vi "simulation.vi"(0 "Angle":dbl[](array[numeric]), 1 "dt":dbl=0.01, 2 "Map Data":T1, 5 "R dir":dbl(slide) scale=3.2..-3.2, 7 "Robot Radius":dbl=6.0, 9 "R pos":dbl[](array[numeric])=[0.0, 0.0], 11 "LRF range":dbl=40.0, 12 "w":dbl=2.0, 13 "LRF offset":dbl=5.0, 14 "v":dbl=2.0) -> (3 "Mapped Data Visual out":T2(graph), 4 "Robot pos new":dbl[](array[numeric]), 10 "Robot dir new":dbl(slide) scale=3.2..-3.2, 15 "LRF":dbl[](array[numeric]))   [LabVIEW 2009]
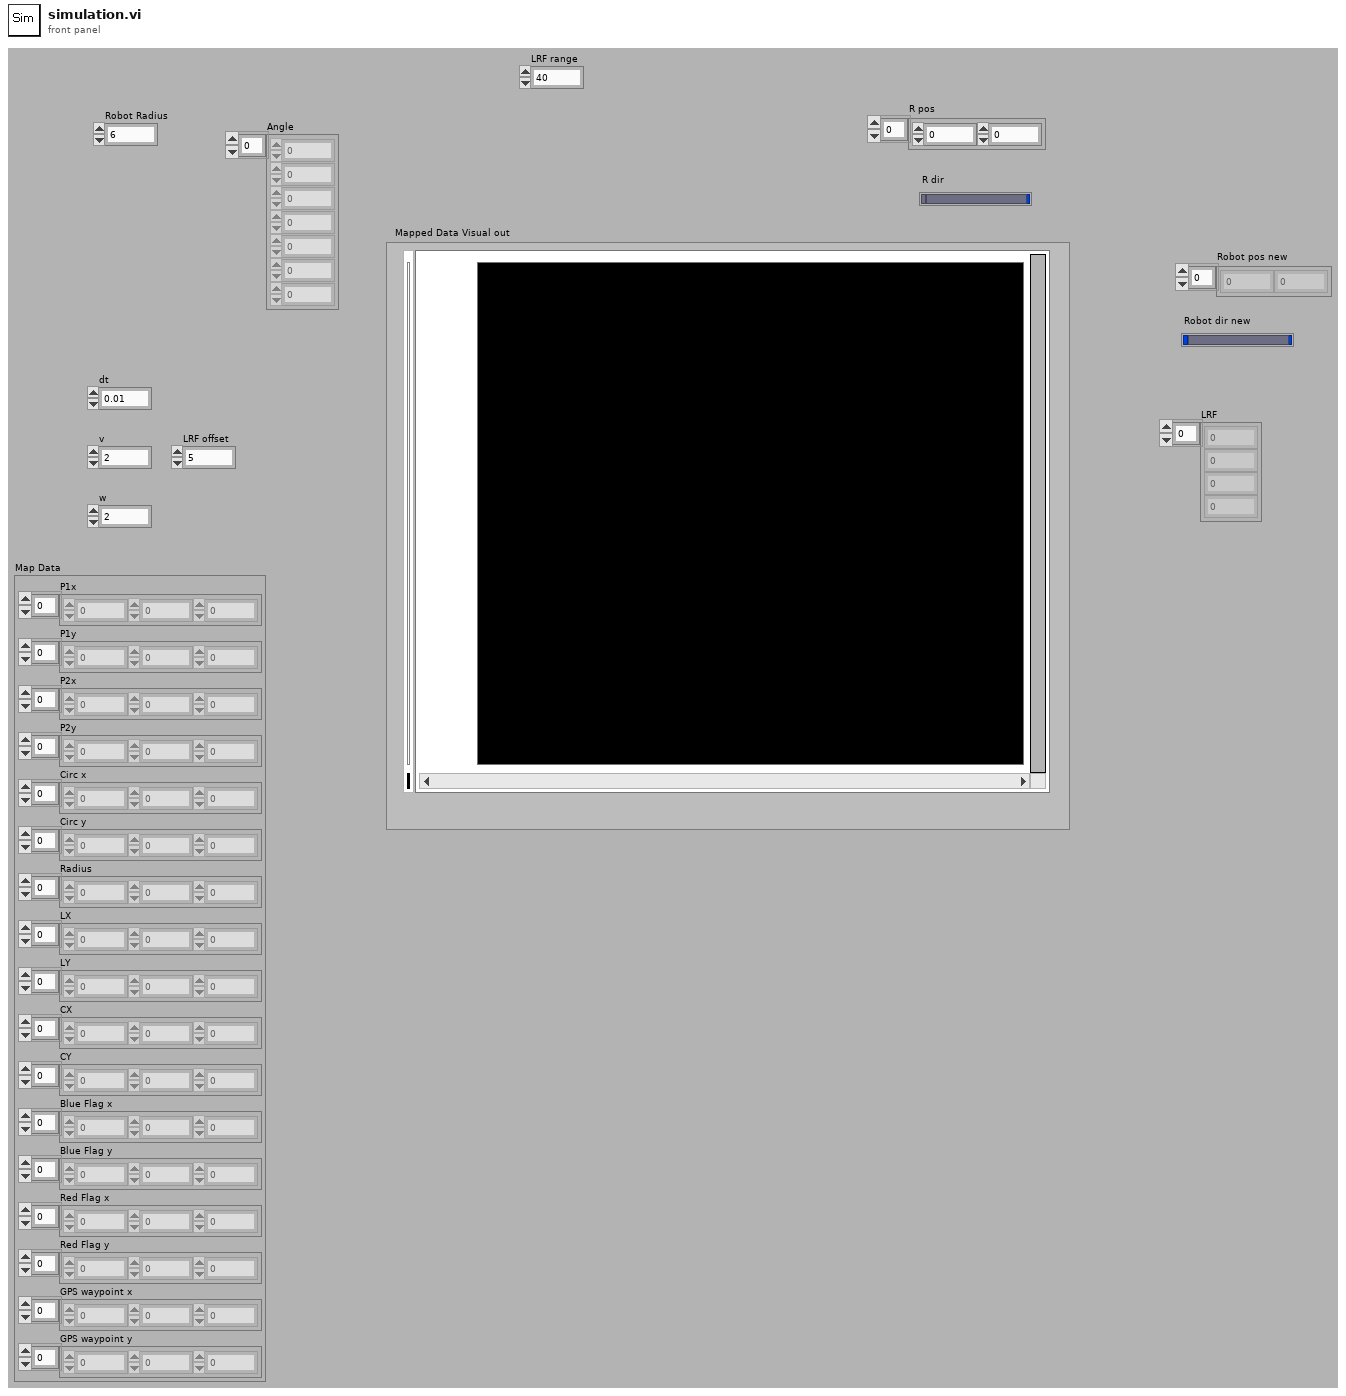
[diagram p1: front panel]
types:
  T1 = cluster{"P1x":dbl[], "P1y":dbl[], "P2x":dbl[], "P2y":dbl[], "Circ x":dbl[], "Circ y":dbl[], "Radius":dbl[], "LX":dbl[], "LY":dbl[], "CX":dbl[], "CY":dbl[], "Blue Flag x":dbl[], "Blue Flag y":dbl[], "Red Flag x":dbl[], "Red Flag y":dbl[], "GPS waypoint x":dbl[], "GPS waypoint y":dbl[]}
  T2 = cluster{cluster{dbl[], dbl[]}, "output cluster":cluster{dbl[], dbl[]}, cluster{dbl[], dbl[]}, cluster{dbl[], dbl[]}, cluster{dbl[], dbl[]}, cluster{dbl[], dbl[]}, cluster{dbl[], dbl[]}}
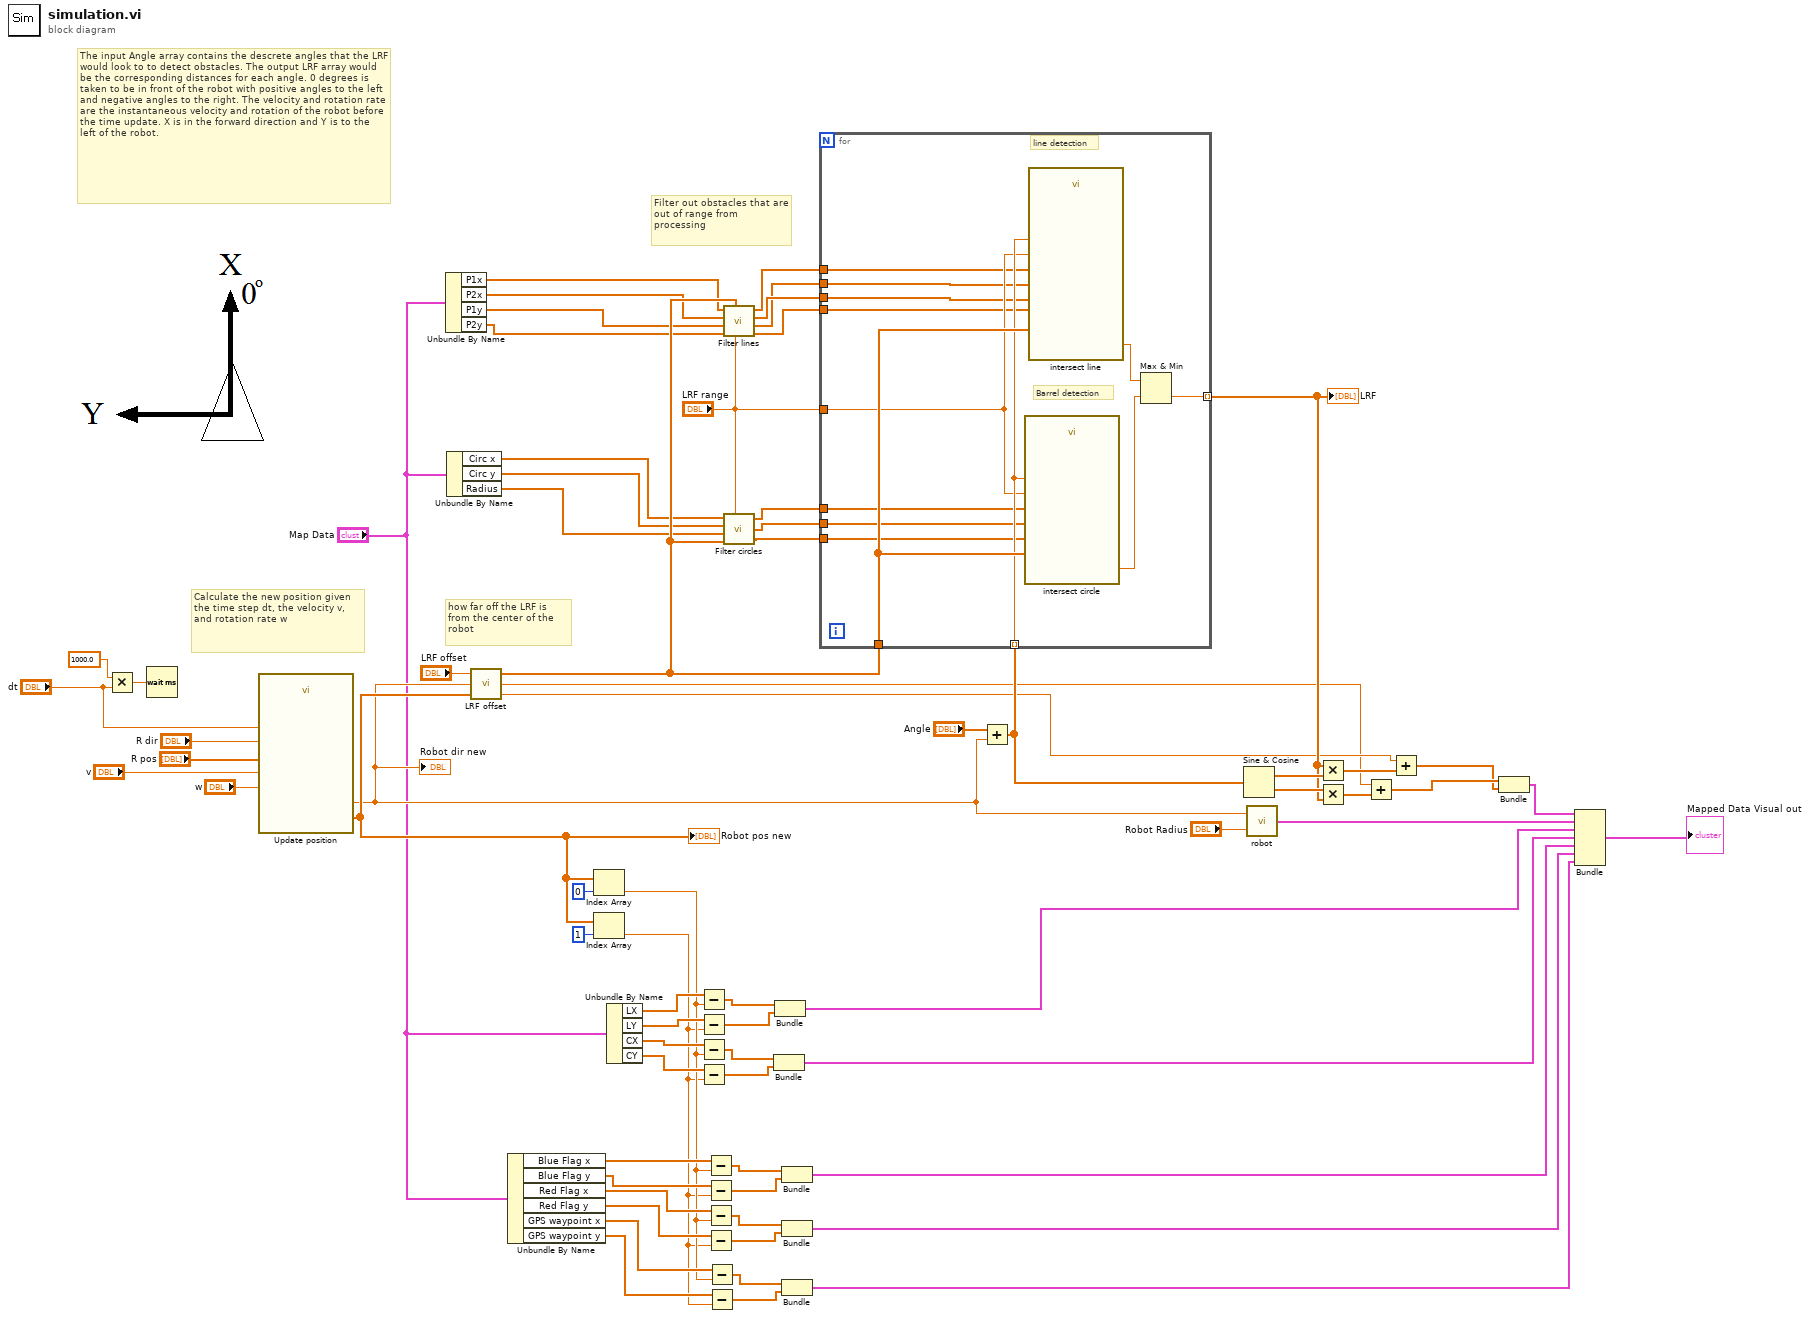
[diagram p0: block diagram]
diagram:
  # "how far off the LRF is from the center of the robot"
  # "The input Angle array contains the descrete angles that the LRF would look to to detect obstacles. The output LRF array would be the corresponding distances for each angle. 0 degrees is taken to be in front of the robot with positive angles to the left and negative angles to the right. The velocity and rotation rate are the instantaneous velocity and rotation of the robot before the time update. X is in the forward direction and Y is to the left of the robot."
  # "Filter out obstacles that are out of range from processing"
  # "Calculate the new position given the time step dt, the velocity v, and rotation rate w"
  n1 = Multiply(x=1000.0 ("y"), y="dt") -> (x*y=w66:dbl)
  n2 = Wait (ms)(milliseconds to wait=w66) -> ()  [unwired: 1 out]
  n3 = call "Update position.vi"("R pos"="R pos", "R dir"="R dir", "dt"="dt", "v"="v", "w"="w") -> ("R pos new"=w30:dbl[], "R dir new"=w20:dbl)
  "Robot pos new" <- w30
  "Robot dir new" <- w20
  n4 = Unbundle By Name("Map Data") -> ("P1x"=w37:dbl[], "P2x"=w36:dbl[], "P1y"=w35:dbl[], "P2y"=w34:dbl[])
  n5 = Unbundle By Name("Map Data") -> ("Circ x"=w40:dbl[], "Circ y"=w39:dbl[], "Radius"=w38:dbl[])
  n6 = call "LRF offset.vi"("Robot position"=w30, "Robot direction"=w20, "LRF offset"="LRF offset") -> ("Dy"=w43:dbl, "Dx"=w42:dbl, "LRF position"=w47:dbl[])
  n7 = Unbundle By Name("Map Data") -> ("Blue Flag x"=w15:dbl[], "Blue Flag y"=w14:dbl[], "Red Flag x"=w13:dbl[], "Red Flag y"=w12:dbl[], "GPS waypoint x"=w9:dbl[], "GPS waypoint y"=w8:dbl[])
  n8 = Index Array(array=w30, index=0) -> (element=w7:dbl)
  n9 = Index Array(array=w30, index=1) -> (element=w6:dbl)
  n10 = Unbundle By Name("Map Data") -> ("LX"=w33:dbl[], "LY"=w29:dbl[], "CX"=w28:dbl[], "CY"=w27:dbl[])
  n11 = Subtract(x=w33, y=w7) -> (x-y=w26:dbl[])
  n12 = Subtract(x=w29, y=w6) -> (x-y=w25:dbl[])
  n13 = Subtract(x=w28, y=w7) -> (x-y=w24:dbl[])
  n14 = Subtract(x=w27, y=w6) -> (x-y=w23:dbl[])
  n15 = Subtract(x=w15, y=w7) -> (x-y=w19:dbl[])
  n16 = Subtract(x=w14, y=w6) -> (x-y=w18:dbl[])
  n17 = Subtract(x=w13, y=w7) -> (x-y=w17:dbl[])
  n18 = Subtract(x=w12, y=w6) -> (x-y=w16:dbl[])
  n19 = Subtract(x=w9, y=w7) -> (x-y=w11:dbl[])
  n20 = Subtract(x=w8, y=w6) -> (x-y=w10:dbl[])
  n21 = call "Filter lines.vi"("max dist"="LRF range", "LRF pos"=w47, "P2y"=w34, "P1y"=w35, "P2x"=w36, "P1x"=w37) -> ("P2y new"=w53:dbl[], "P1y new"=w54:dbl[], "P2x new"=w55:dbl[], "P1x new"=w56:dbl[])
  n22 = call "Filter circles.vi"("Circ x"=w40, "Circ y"=w39, "R"=w38, "LRF pos"=w47, "max dist"="LRF range") -> ("Circ x out"=w51:dbl[], "Circ y out"=w50:dbl[], "R out"=w49:dbl[])
  n23 = Bundle(w24, w23) -> (w21:cluster{dbl[], dbl[]})  [unwired: 1 in]
  n24 = Bundle(w26, w25) -> (w22:cluster{dbl[], dbl[]})  [unwired: 1 in]
  n25 = Bundle(w19, w18) -> (w5:cluster{dbl[], dbl[]})  [unwired: 1 in]
  n26 = Bundle(w17, w16) -> (w4:cluster{dbl[], dbl[]})  [unwired: 1 in]
  n27 = Bundle(w11, w10) -> (w3:cluster{dbl[], dbl[]})  [unwired: 1 in]
  n28 = Add(x="Angle", y=w20) -> (x+y=w67:dbl[])
  n29 = for {
    tunnel: w67 -> [w80] mode=indexing
    tunnel: [w81] -> w69 mode=indexing
    tunnel: w47 -> [w84]
    tunnel: "LRF range" -> [w79]
    tunnel: w56 -> [w78]
    tunnel: w55 -> [w77]
    tunnel: w54 -> [w76]
    tunnel: w53 -> [w75]
    tunnel: w51 -> [w74]
    tunnel: w50 -> [w73]
    tunnel: w49 -> [w72]
    # "line detection"
    # "Barrel detection"
    n30 = call "intersect circle.vi"("max dist"=w79, "R"=w72, "Look"=w80, "R pos"=w84, "py"=w73, "px"=w74) -> ("Dist"=w83:dbl)
    n31 = call "intersect line.vi"("R pos"=w84, "max dist"=w79, "look dir"=w80, "P2y"=w75, "P2x"=w77, "P1y"=w76, "P1x"=w78) -> ("Dist"=w82:dbl)
    n32 = Max & Min(x=w82, y=w83) -> (min(x,y)=w81:dbl)  [unwired: 1 out]
  }
  "LRF" <- w69
  n33 = Sine & Cosine(0:w67) -> (1:w71:dbl[], 2:w70:dbl[])
  n34 = call "robot.vi"("Robot Radius"="Robot Radius", "direction"=w20) -> ("output cluster"=w58:cluster{dbl[], dbl[]})
  n35 = Multiply(x=w69, y=w71) -> (x*y=w44:dbl[])
  n36 = Multiply(x=w70, y=w69) -> (x*y=w41:dbl[])
  n37 = Add(x=w42, y=w41) -> (x+y=w46:dbl[])
  n38 = Add(x=w43, y=w44) -> (x+y=w45:dbl[])
  n39 = Bundle(w46, w45) -> (w57:cluster{dbl[], dbl[]})  [unwired: 1 in]
  n40 = Bundle(w57, "output cluster"=w58, w22, w21, w5, w4, w3) -> (→"Mapped Data Visual out":T2)  [unwired: 1 in]
